vi "Globals to XML.vi"(8 "Array":path[](array[path])) -> ()   [LabVIEW 2020]
uses:
  <vilib>/Utility/xml.llb/Write to XML File(string).vi
  Globals/Turret_Globals.vi
  Globals/Flywheel_Globals.vi
  Globals/Feeder_Globals.vi
  Globals/Drive_Globals.vi
  Globals/Cowl_Globals.vi
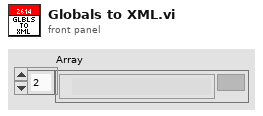
[diagram p1: front panel]
types:
  T1 = cluster{"Turret_Kd":dbl, "Turret_Ki":dbl, "Turret_Kd":dbl, "Turret_Lower_Limit_Value":dbl, "Turret_Upper_Limit_Value":dbl}
  T2 = cluster{"Magazine_Firing_Velocity":dbl, "Magazine_Load_%Vbus":dbl}
  T3 = cluster{"Min Output":dbl, "Max Ouput":dbl, "Int Error Window":dbl, "N-Int":i32, "N-Diff":i32, "Kd":dbl, "Ki":dbl, "Kp":dbl}
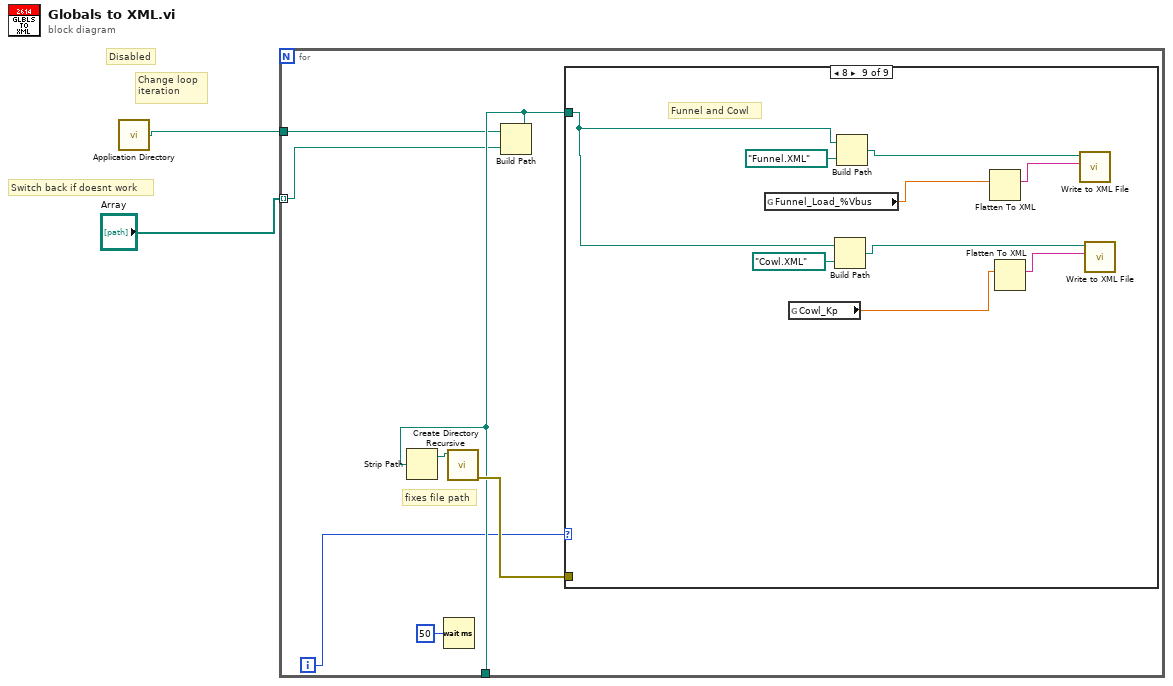
[diagram p0: block diagram]
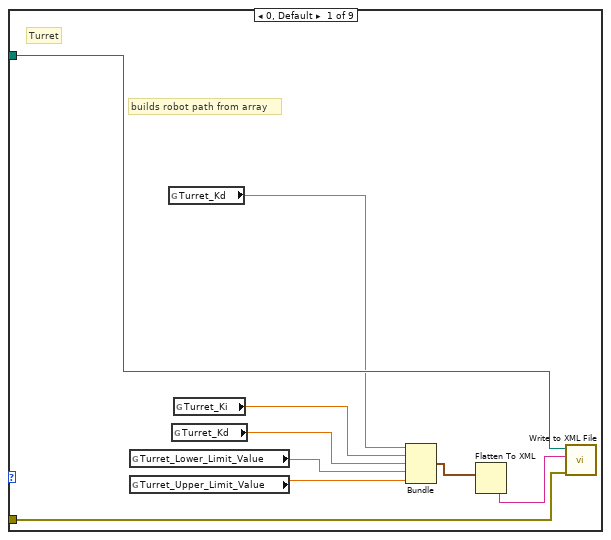
[diagram p2: hidden frame]
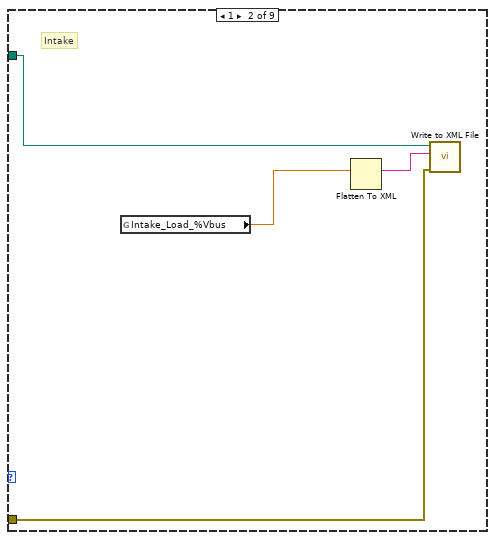
[diagram p3: hidden frame]
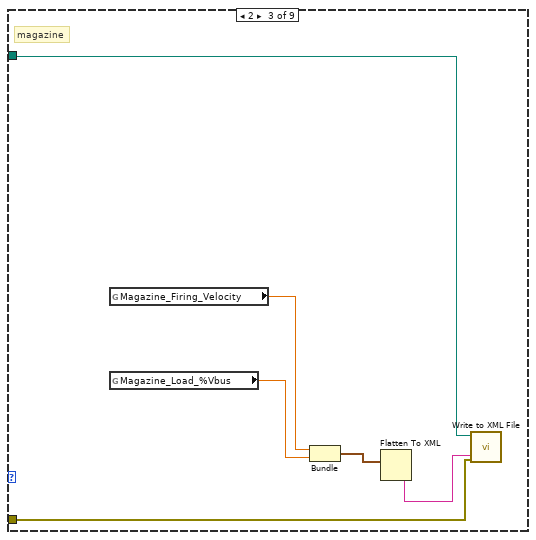
[diagram p4: hidden frame]
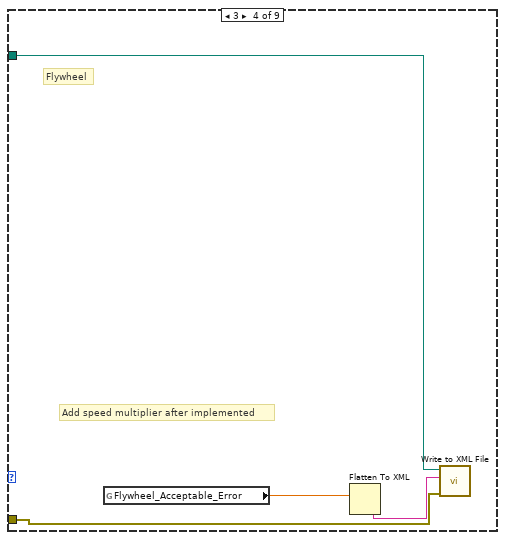
[diagram p5: hidden frame]
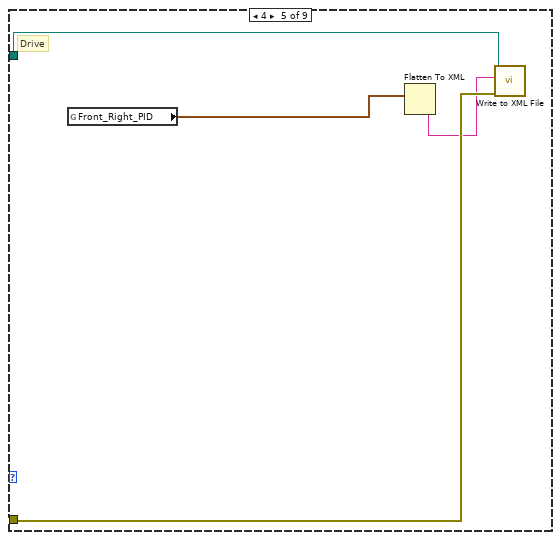
[diagram p6: hidden frame]
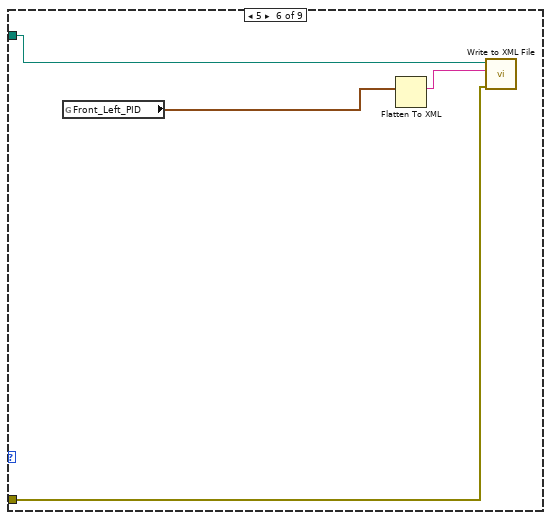
[diagram p7: hidden frame]
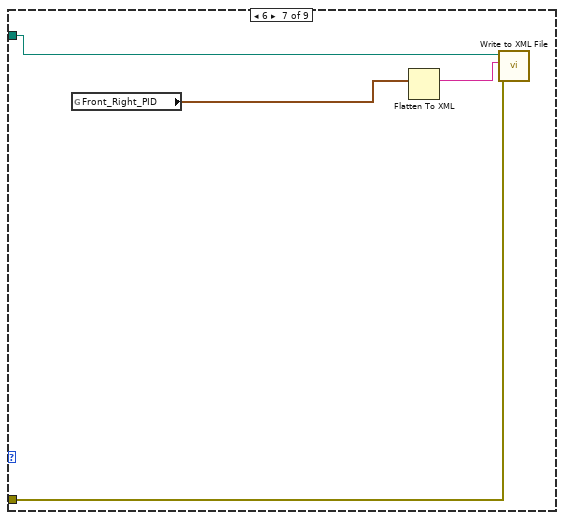
[diagram p8: hidden frame]
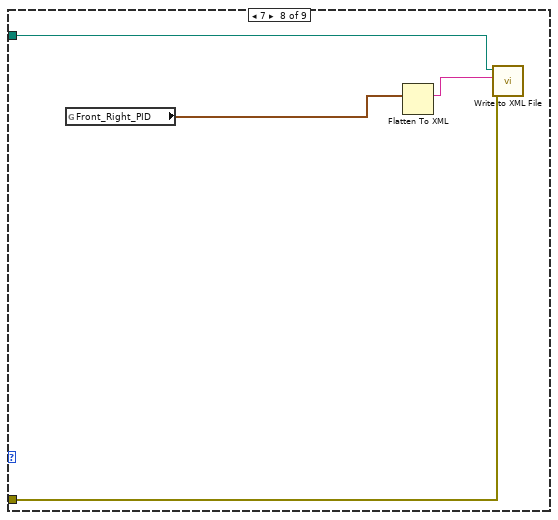
[diagram p9: hidden frame]
diagram:
  # "Switch back if doesnt work"
  # "Change loop\niteration"
  # "Disabled"
  n1 = call <vilib>:"Application Directory.vi"() -> ("Application Directory"=w2:path)
  n2 = for {
    tunnel: [w6] -> _
    tunnel: w2 -> [w5]
    tunnel: "Array" -> [w4] mode=indexing
    i -> [w3]
    # "fixes file path"
    n3 = Wait (ms)(milliseconds to wait=u32 50) -> ()  [unwired: 1 out]
    n4 = Build Path(base path=w5, name or relative path=w4) -> (appended path=w6:path)
    n5 = Strip Path(path=w6) -> (stripped path=w8:path)  [unwired: 1 out]
    n6 = call <vilib>:"Create Directory Recursive.vi"("directory"=w8) -> ("error out"=w7:errorcluster)  [unwired: 4 in, 2 out]
    n7 = case shown="8" w3 {
      tunnel: w6 -> [w17 w22 w26 w32 w36 w39 w43 w47 w55]
      tunnel: w7 -> [w16 w21 w25 w31 w35 w37 w41 w46 _]
      frame 0, Default {
        # "builds robot path from array"
        # "Turret"
        n8 = global read "Turret_Globals.vi" "Turret_Lower_Limit_Value"() -> (w11:dbl)
        n9 = global read "Turret_Globals.vi" "Turret_Upper_Limit_Value"() -> (w10:dbl)
        n10 = global read "Turret_Globals.vi" "Turret_Kd"() -> (w14:dbl)
        n11 = global read "Turret_Globals.vi" "Turret_Kd"() -> (w12:dbl)
        n12 = global read "Turret_Globals.vi" "Turret_Ki"() -> (w13:dbl)
        n13 = Bundle("Turret_Kd"=w14, "Turret_Ki"=w13, "Turret_Kd"=w12, "Turret_Lower_Limit_Value"=w11, "Turret_Upper_Limit_Value"=w10) -> (w18:T1)  [unwired: 1 in]
        n14 = Flatten To XML(anything=w18) -> (xml string=w15:string)
        n15 = call-poly <vilib>:"Write to XML File.vi"("error in (no error)"=w16, "XML Input"=w15, "XML File Path"=w17) -> ()  [unwired: 6 in, 3 out]
      }
      frame 1 {
        # "Intake"
        n16 = global read "Feeder_Globals.vi" "Intake_Load_%Vbus"() -> (w19:dbl)
        n17 = Flatten To XML(anything=w19) -> (xml string=w20:string)
        n18 = call-poly <vilib>:"Write to XML File.vi"("error in (no error)"=w21, "XML Input"=w20, "XML File Path"=w22) -> ()  [unwired: 6 in, 3 out]
      }
      frame 2 {
        # "magazine"
        n19 = global read "Feeder_Globals.vi" "Magazine_Firing_Velocity"() -> (w24:dbl)
        n20 = global read "Feeder_Globals.vi" "Magazine_Load_%Vbus"() -> (w23:dbl)
        n21 = Bundle("Magazine_Firing_Velocity"=w24, "Magazine_Load_%Vbus"=w23) -> (w27:T2)  [unwired: 1 in]
        n22 = Flatten To XML(anything=w27) -> (xml string=w28:string)
        n23 = call-poly <vilib>:"Write to XML File.vi"("error in (no error)"=w25, "XML Input"=w28, "XML File Path"=w26) -> ()  [unwired: 6 in, 3 out]
      }
      frame 3 {
        # "Add speed multiplier after implemented"
        # "Flywheel"
        n24 = global read "Flywheel_Globals.vi" "Flywheel_Acceptable_Error"() -> (w29:dbl)
        n25 = Flatten To XML(anything=w29) -> (xml string=w30:string)
        n26 = call-poly <vilib>:"Write to XML File.vi"("error in (no error)"=w31, "XML Input"=w30, "XML File Path"=w32) -> ()  [unwired: 6 in, 3 out]
      }
      frame 4 {
        # "Drive"
        n27 = global read "Drive_Globals.vi" "Front_Right_PID"() -> (w33:T3)
        n28 = Flatten To XML(anything=w33) -> (xml string=w34:string)
        n29 = call-poly <vilib>:"Write to XML File.vi"("error in (no error)"=w35, "XML Input"=w34, "XML File Path"=w36) -> ()  [unwired: 6 in, 3 out]
      }
      frame 5 {
        n30 = global read "Drive_Globals.vi" "Front_Left_PID"() -> (w40:T3)
        n31 = Flatten To XML(anything=w40) -> (xml string=w38:string)
        n32 = call-poly <vilib>:"Write to XML File.vi"("error in (no error)"=w37, "XML Input"=w38, "XML File Path"=w39) -> ()  [unwired: 6 in, 3 out]
      }
      frame 6 {
        n33 = global read "Drive_Globals.vi" "Front_Right_PID"() -> (w44:T3)
        n34 = Flatten To XML(anything=w44) -> (xml string=w42:string)
        n35 = call-poly <vilib>:"Write to XML File.vi"("error in (no error)"=w41, "XML Input"=w42, "XML File Path"=w43) -> ()  [unwired: 6 in, 3 out]
      }
      frame 7 {
        n36 = global read "Drive_Globals.vi" "Front_Right_PID"() -> (w48:T3)
        n37 = Flatten To XML(anything=w48) -> (xml string=w45:string)
        n38 = call-poly <vilib>:"Write to XML File.vi"("error in (no error)"=w46, "XML Input"=w45, "XML File Path"=w47) -> ()  [unwired: 6 in, 3 out]
      }
      frame 8 {
        # "Funnel and Cowl"
        n39 = global read "Feeder_Globals.vi" "Funnel_Load_%Vbus"() -> (w50:dbl)
        n40 = global read "Cowl_Globals.vi" "Cowl_Kp"() -> (w49:dbl)
        n41 = Build Path(base path=w55, name or relative path=path "/Cowl.XML") -> (appended path=w51:path)
        n42 = Build Path(base path=w55, name or relative path=path "/Funnel.XML") -> (appended path=w52:path)
        n43 = Flatten To XML(anything=w50) -> (xml string=w57:string)
        n44 = Flatten To XML(anything=w49) -> (xml string=w56:string)
        n45 = call-poly <vilib>:"Write to XML File.vi"("XML Input"=w57, "XML File Path"=w52) -> ()  [unwired: 7 in, 3 out]
        n46 = call-poly <vilib>:"Write to XML File.vi"("XML Input"=w56, "XML File Path"=w51) -> ()  [unwired: 7 in, 3 out]
      }
    }
  }
